vi "sub_chart_pie.vi"(0 "CHART REF IN":refnum<vi>, 1 "TITLE":string, 3 "DATA":T1, 5 "ERROR IN":errorcluster) -> (14 "CHART REF OUT":refnum<vi>, 17 "CHART":picture, 19 "ERROR OUT":errorcluster)   [LabVIEW 2018]
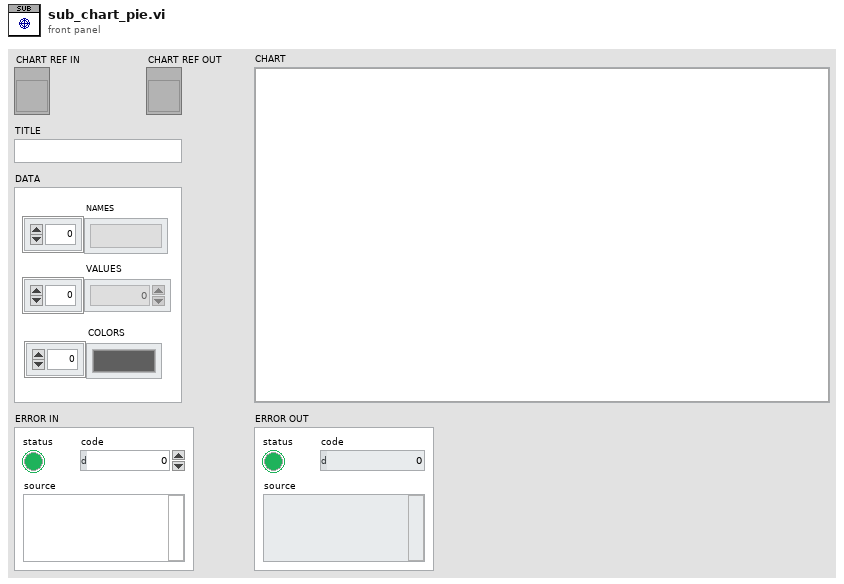
[diagram p1: front panel]
types:
  T1 = cluster{"NAMES":string[], "VALUES":dbl[], "COLORS":u32[]}
  T2 = enum16{"User-specified Font", "Application Font", "System Font", "Dialog Font"}
  T3 = cluster{"Font Name:":string, "Size":i16, "Strikeout?":bool, "Italic?":bool, "Underline?":bool, "Outline?":bool, "Shadow?":bool, "Bold?":bool}
  T4 = enum32{"Bad", "Idle", "Run top level", "Running"}
  T5 = typedef "LVBoundsTypeDef.ctl" = cluster{"Width":u32, "Height":u32}
  T6 = cluster{"left":i16, "top":i16, "right":i16, "bottom":i16}
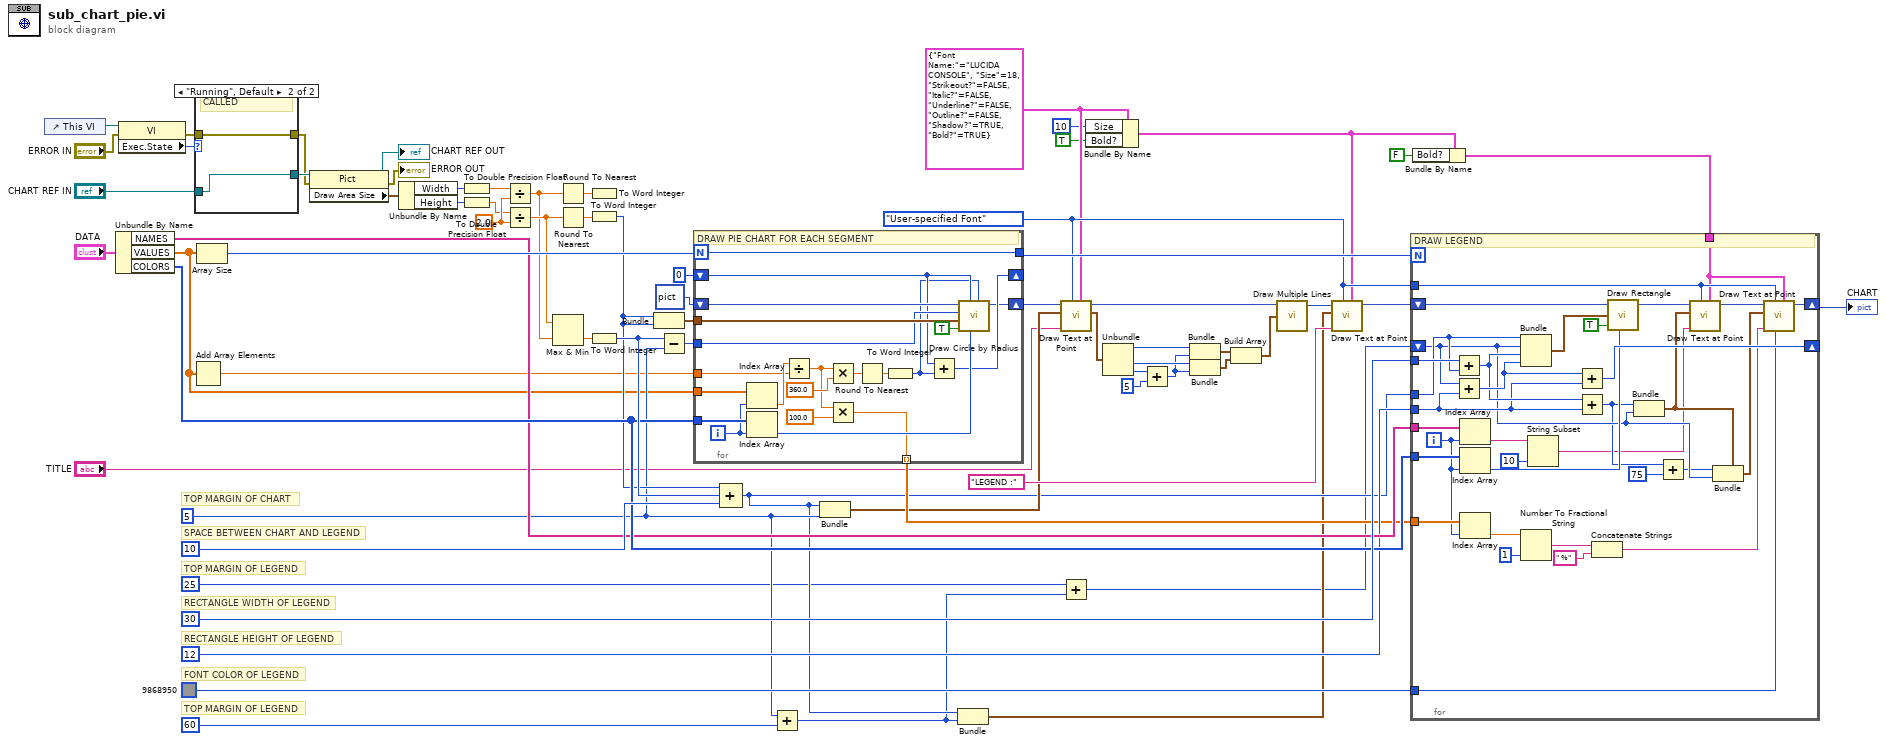
[diagram p0: block diagram]
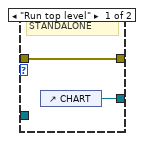
[diagram p2: hidden frame]
diagram:
  w24 = T2."User-specified Font" ("desired font(Application)")
  w23 = T3 {"Font Name:"="LUCIDA CONSOLE", "Size"=18, "Strikeout?"=FALSE, "Italic?"=FALSE, "Underline?"=FALSE, "Outline?"=FALSE, "Shadow?"=TRUE, "Bold?"=TRUE} ("[user-specified font]")
  w30 = i16 5 ("y")
  w61 = 2.0 ("y")
  # "TOP MARGIN OF LEGEND"
  # "FONT COLOR OF LEGEND"
  # "RECTANGLE HEIGHT OF LEGEND"
  # "RECTANGLE WIDTH OF LEGEND"
  # "TOP MARGIN OF LEGEND"
  # "SPACE BETWEEN CHART AND LEGEND"
  # "TOP MARGIN OF CHART"
  n1 = control-ref of="This VI"() -> (w69:refnum<vi>)
  n2 = Unbundle By Name("DATA") -> ("NAMES"=w38:string[], "VALUES"=w3:dbl[], "COLORS"=w40:u32[])
  n3 = property class="VI"(reference=w69, error in="ERROR IN") -> (error out=w7:errorcluster, "Exec.State"=w68:T4)  [unwired: 1 out]
  n4 = Add Array Elements(numeric array=w3) -> (sum=w2:dbl)
  n5 = case shown="\"Running\", Default" w68 {
    tunnel: [w71 w73] -> w67
    tunnel: "CHART REF IN" -> [_ w73]
    tunnel: w7 -> [w70 w72]
    tunnel: [w70 w72] -> w6
    frame "Run top level" {
      # "STANDALONE"
      n6 = control-ref of="CHART"() -> (w71:refnum<vi>)
    }
    frame "Running", Default {
      # "CALLED"
    }
  }
  n7 = Array Size(array=w3) -> (size(s)=w63:i32)
  n8 = property class="Pict"(reference=w67, error in=w6) -> (reference out=→"CHART REF OUT":refnum<vi>, error out=→"ERROR OUT":errorcluster, "Draw Area Size"=w65:T5)
  n9 = Unbundle By Name(w65) -> ("Width"=w55:u32, "Height"=w56:u32)
  n10 = To Double Precision Float(number=w55) -> (double precision float=w62:dbl)
  n11 = To Double Precision Float(number=w56) -> (double precision float=w57:dbl)
  n12 = Divide(x=w62, y=w61) -> (x/y=w51:dbl)
  n13 = Divide(x=w57, y=w61) -> (x/y=w52:dbl)
  n14 = Max & Min(x=w52, y=w51) -> (min(x,y)=w53:dbl)  [unwired: 1 out]
  n15 = Round To Nearest(number=w51) -> (nearest integer value=w60:dbl)
  n16 = Round To Nearest(number=w52) -> (nearest integer value=w59:dbl)
  n17 = To Word Integer(number=w60) -> ()  [unwired: 1 out]
  n18 = To Word Integer(number=w59) -> (16bit integer=w34:i16)
  n19 = To Word Integer(number=w53) -> (16bit integer=w47:i16)
  n20 = Bundle(w34, w34) -> (w58:cluster{i16, i16})  [unwired: 1 in]
  n21 = Subtract(x=w47, y=w30) -> (x-y=w49:i16)
  n22 = for {
    N: w63 -> [w78]
    tunnel: w58 -> [w94]
    tunnel: w49 -> [w92]
    tunnel: w40 -> [w91]
    tunnel: w3 -> [w88]
    shift-right: [w80] -> _
    shift-left: i16 0 -> [w81]
    tunnel: w2 -> [w82]
    shift-right: [w77] -> w33
    shift-left: picture data[5B] ("new picture") -> [w84]
    tunnel: [w78] -> w45
    tunnel: [w74] -> w36 mode=indexing
    i -> [w89]
    # "DRAW PIE CHART FOR EACH SEGMENT"
    n23 = Index Array(array=w88, index=w89) -> (element=w83:dbl)
    n24 = Index Array(array=w91, index=w89) -> (element=w90:u32)
    n25 = Divide(x=w83, y=w82) -> (x/y=w76:dbl)
    n26 = Multiply(x=w76, y=360.0) -> (x*y=w86:dbl)
    n27 = Multiply(x=w76, y=100.0) -> (x*y=w74:dbl)
    n28 = Round To Nearest(number=w86) -> (nearest integer value=w85:dbl)
    n29 = To Word Integer(number=w85) -> (16bit integer=w79:i16)
    n30 = Add(x=w81, y=w79) -> (x+y=w80:i16)
    n31 = call <vilib>:"Draw Circle by Radius.vi"("arc size(360)"=w79, "color(black)"=w90, "start angle(0)"=w81, "fill?(F)"=TRUE, "pixel center"=w94, "radius"=w92, "picture"=w84) -> ("new picture"=w77:picture)  [unwired: 4 in]
  }
  n32 = Compound Arithmetic op=ADD(w34, w47, i16 10 ("value")) -> (w29:i16)
  n33 = Add(x=w30, y=i16 60) -> (x+y=w27:i16)
  n34 = Bundle(w29, "y"=w30) -> (w32:cluster{i16, "y":i16})  [unwired: 1 in]
  n35 = Bundle(w29, w27) -> (w28:cluster{i16, i16})  [unwired: 1 in]
  n36 = call <vilib>:"Draw Text at Point.vi"("[user-specified font]"=w23, "desired font(Application)"=w24, "text"="TITLE", "origin"=w32, "picture"=w33) -> ("text rect"=w17:T6, "new picture"=w19:picture)  [unwired: 5 in]
  n37 = Add(x=i16 25, y=w27) -> (x+y=w26:i16)
  n38 = Bundle By Name(cluster=w23, "Size"=i16 10, "Bold?"=TRUE) -> (w20:T3)
  n39 = Unbundle(w17) -> ("left"=w14:i16, "right"=w11:i16, "bottom"=w12:i16)  [unwired: 1 out]
  n40 = Add(x=w12, y=i16 5) -> (x+y=w9:i16)
  n41 = Bundle("left"=w14, w9) -> (w16:cluster{"left":i16, i16})  [unwired: 1 in]
  n42 = Bundle("right"=w11, w9) -> (w10:cluster{"right":i16, i16})  [unwired: 1 in]
  n43 = Build Array(w16, w10) -> (w15:cluster{"right":i16, i16}[])
  n44 = call <vilib>:"Draw Multiple Lines.vi"("picture"=w19, "line endpoints"=w15) -> ("new picture"=w18:picture)  [unwired: 7 in]
  n45 = call <vilib>:"Draw Text at Point.vi"("[user-specified font]"=w20, "desired font(Application)"=w24, "text"="LEGEND :", "origin"=w28, "picture"=w18) -> ("new picture"=w44:picture)  [unwired: 5 in, 1 out]
  n46 = Bundle By Name(cluster=w20, "Bold?"=FALSE) -> (w41:T3)
  n47 = for {
    N: w45 -> [_]
    tunnel: w38 -> [w128]
    shift-right: [w125] -> _
    shift-left: w26 -> [w106]
    tunnel: i16 30 -> [w119]
    tunnel: w40 -> [w123]
    shift-right: [w110] -> w35
    shift-left: w44 -> [w127]
    tunnel: u32 9868950 -> [w99]
    tunnel: w24 -> [w109]
    tunnel: w41 -> [w95]
    tunnel: w29 -> [w118]
    tunnel: i16 12 ("y") -> [w116]
    tunnel: w36 -> [w115]
    i -> [w114]
    # "DRAW LEGEND"
    n48 = Add(x=w119, y=w118) -> (x+y=w117:i16)
    n49 = Add(x=w106, y=w116) -> (x+y=w126:i16)
    n50 = Index Array(array=w128, index=w114) -> (element=w98:string)
    n51 = Index Array(array=w123, index=w114) -> (element=w122:u32)
    n52 = Index Array(array=w115, index=w114) -> (element=w113:dbl)
    n53 = Bundle(w118, w106, w117, w126) -> (w120:cluster{i16, i16, i16, i16})  [unwired: 1 in]
    n54 = Number To Fractional String(number=w113, precision (6)=i16 1) -> (F-format string=w102:string)  [unwired: 2 in]
    n55 = String Subset(string=w98, length (rest)=10 ("length (rest)")) -> (substring=w96:string)  [unwired: 1 in]
    n56 = Add(x=w126, y=w116) -> (x+y=w125:i16)
    n57 = Add(x=w117, y=w116) -> (x+y=w105:i16)
    n58 = Concatenate Strings(w102, " %") -> (w100:string)
    n59 = call <vilib>:"Draw Rectangle.vi"("picture"=w127, "rect"=w120, "fill?(F)"=TRUE, "color(black)"=w122) -> ("new picture"=w121:picture)  [unwired: 5 in]
    n60 = Bundle(w105, w106) -> (w108:cluster{i16, i16})  [unwired: 1 in]
    n61 = Add(x=w105, y=i16 75) -> (x+y=w103:i16)
    n62 = call <vilib>:"Draw Text at Point.vi"("[user-specified font]"=w95, "desired font(Application)"=w109, "text"=w96, "origin"=w108, "picture"=w121) -> ("new picture"=w111:picture)  [unwired: 5 in, 1 out]
    n63 = Bundle(cluster=w108, w103, w106) -> (w107:cluster{i16, i16})
    n64 = call <vilib>:"Draw Text at Point.vi"("[user-specified font]"=w95, "text color(black)"=w99, "desired font(Application)"=w109, "text"=w100, "origin"=w107, "picture"=w111) -> ("new picture"=w110:picture)  [unwired: 4 in, 1 out]
  }
  "CHART" <- w35
